vi "ProdaNG.Tree.ProcessStepParams.Add.vi"(5 "Mode":T4, 6 "FileContent":T1, 7 "TestStepsTree":refnum<vi>, 8 "error in (no error)":errorcluster, 9 "units":T5[](array[typedef]), 10 "processStepId":i32, 11 "dbHandleIn":i32) -> (0 "error out":errorcluster, 1 "#changes":i32, 3 "dbHandle":i32)   [LabVIEW 2016]
doc: "This function returns a product structure for a product, which is identified by a part and a serial number.\nImportant information: The field 'individual' was taken over from the field 'allgemein' of the legacy data directly. Because of this most products have the value 0 further on and only a few the value 1. \nParameter:\nhandle is an Integer, which is returned by the function Login() at the creation of a new connection.\nwabcoPartId is the Id of the part.\nserialNumber is the serial number of the product for the part above.\nproduct is a pointer on a product structure, which is filled if the returncode is 0. The structure must be defined in the calling program.\n\nReturncodes:\n0 No error\n< 0 ORACLE Error code\n6 (ERROR_INVALID_HANDLE) in case of an invalid handle\n1403 Record does not exist"
uses:
  Controls/ProdaNG.UnitSimple.ctl
  ProdaNG.Tree.TestViewMode.ctl
  ProdaNG.File.Sequence.ctl
  ProdaNG.Tree.Fglb.Value.ctl
  ProdaNG.File.Step.ctl
  ProdaNG.Tree.Fglb.Data.ctl
  ProdaNG.Tree.Fglb.Element.ctl
  ProdaNG.Tree.Fglb.Action.ctl
  ProdaNG.Configurator.Glb.vi
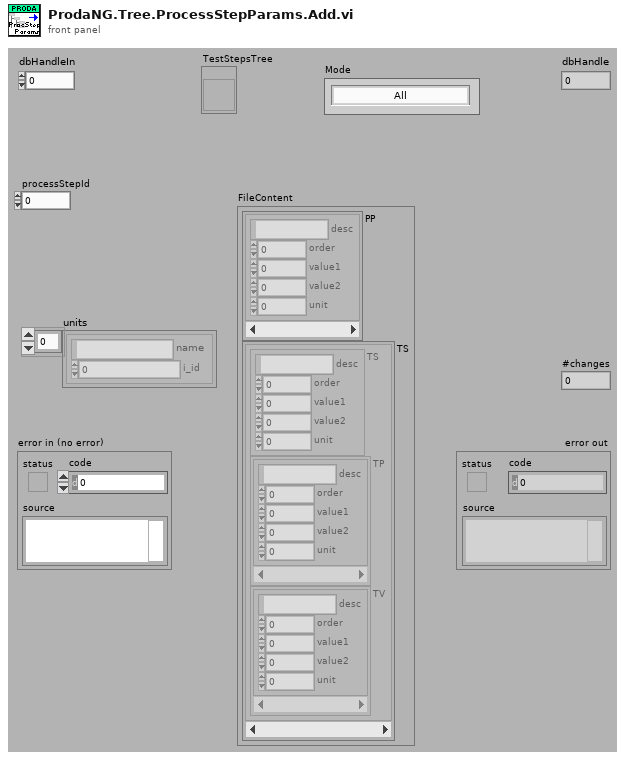
[diagram p1: front panel]
types:
  T1 = typedef "ProdaNG.File.Sequence.ctl" = cluster{"PP":T2[], "TS":T3[]}
  T2 = typedef "ProdaNG.Tree.Fglb.Value.ctl" = cluster{"desc":string, "order":i32, "value1":dbl, "value2":dbl, "unit":i32}
  T3 = typedef "ProdaNG.File.Step.ctl" = cluster{"TS":T2, "TP":T2[], "TV":T2[]}
  T4 = typedef "ProdaNG.Tree.TestViewMode.ctl" = enum16{"All", "Released", "Unreleased"}
  T5 = typedef "ProdaNG.UnitSimple.ctl" = cluster{"name":string, "i_id":i32}
  T6 = typedef "ProdaNG.Tree.Fglb.Action.ctl" = enum16{"init", "add", "get by row", "get by tag", "get by idx"}
  T7 = typedef "ProdaNG.Tree.Fglb.Element.ctl" = enum16{"-", "PP", "TS", "TP", "TV"}
  T8 = typedef "ProdaNG.Tree.Fglb.Data.ctl" = cluster{"tag":string, "row":i32, "element":T7, "idx1":i32, "idx2":i32, "file":bool}
  T9 = typedef "ProdaNG.ProcessStepParam.ctl" = cluster{"i_id":i32, "processStepId":i32, "unitId":i32, "contentId":string, "previewId":string, "value":dbl, "valueText":string, "paramSequence":i32, "history":i32, "mdReason":string, "mdUser":string, "mdTime":string, "description":string}
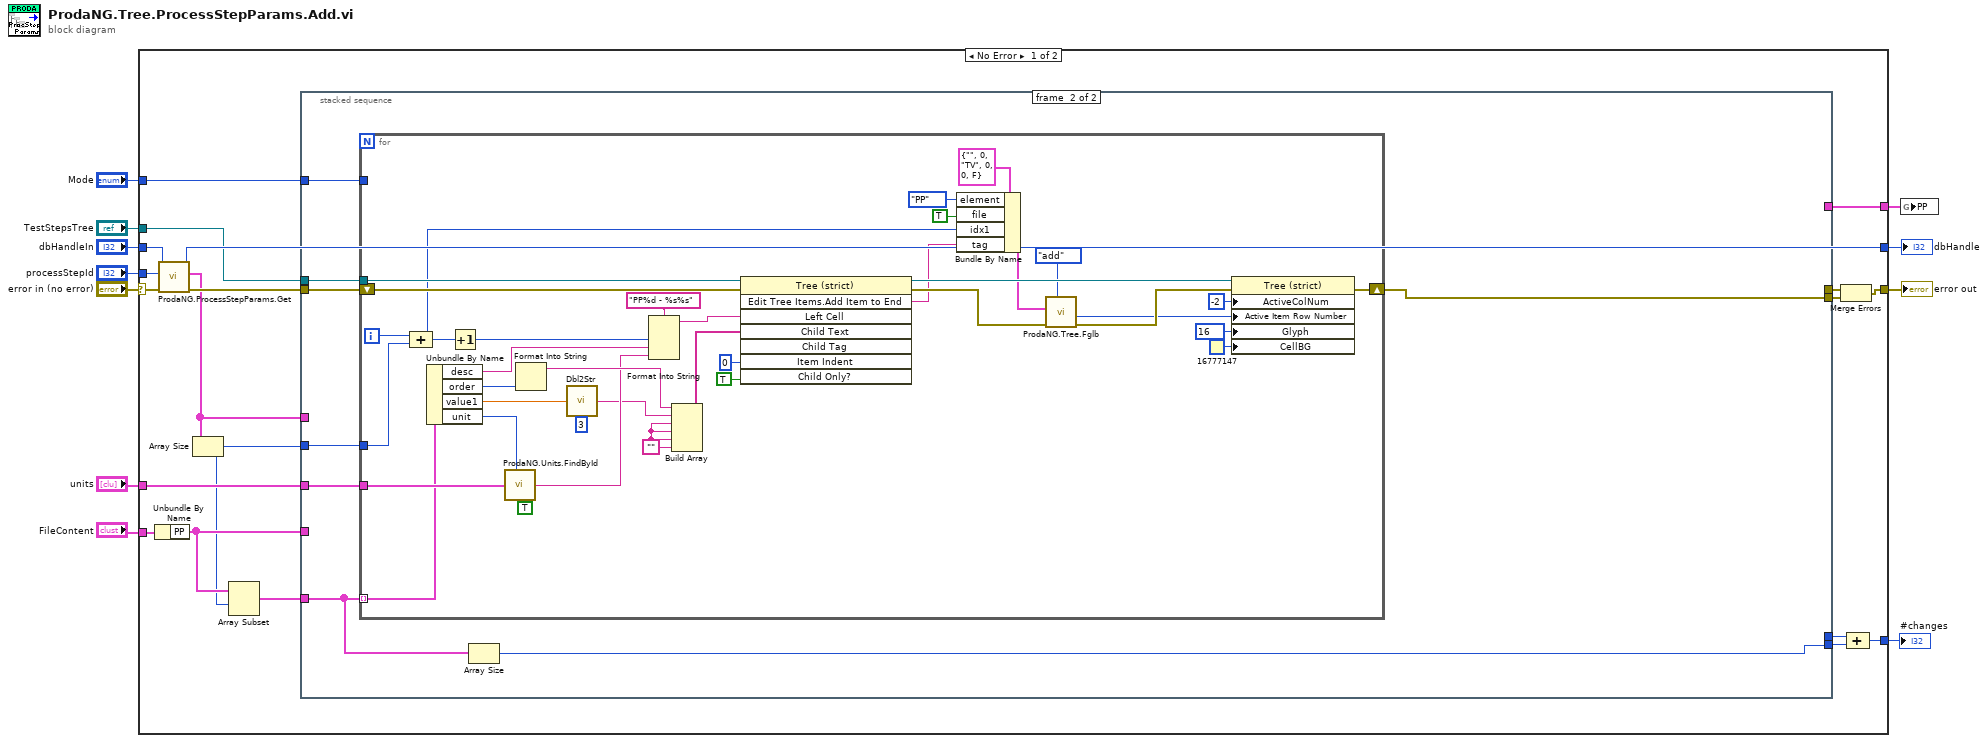
[diagram p0: block diagram]
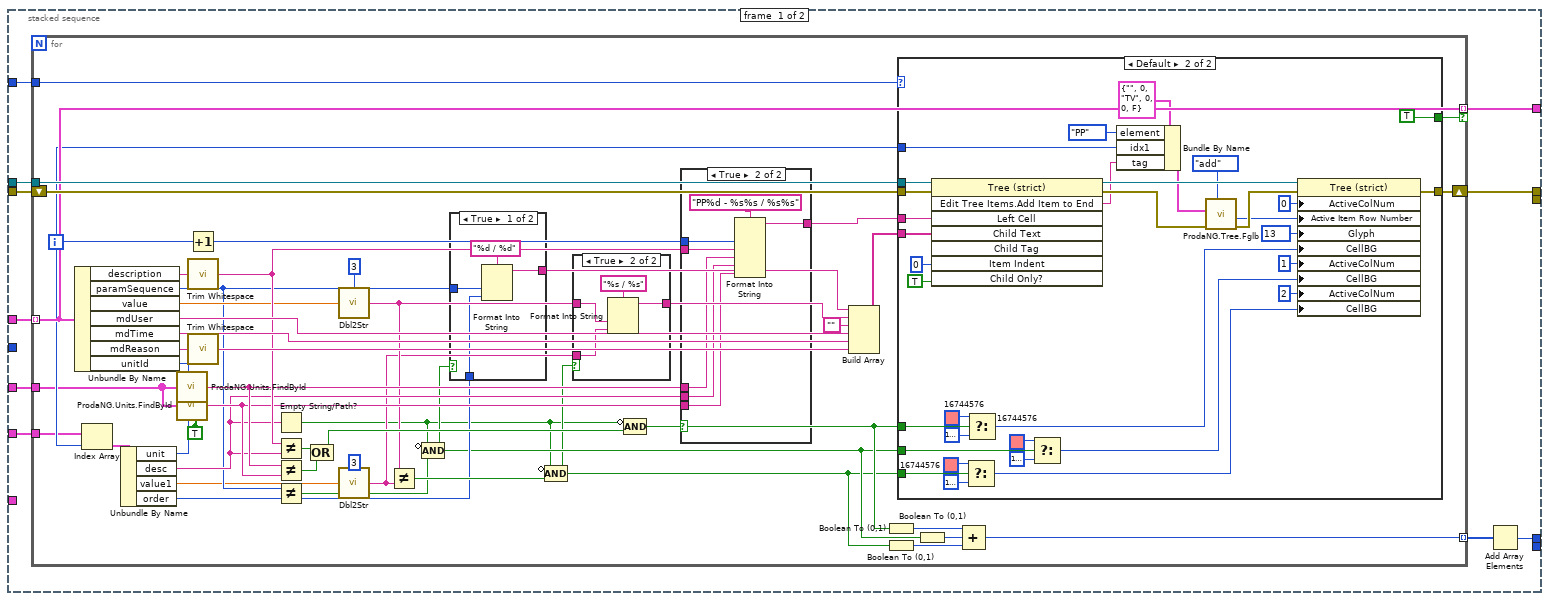
[diagram p2: hidden frame]
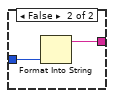
[diagram p3: hidden frame]
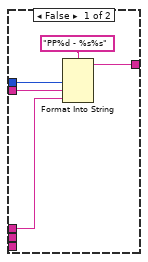
[diagram p5: hidden frame]
diagram:
  n1 = case shown="No Error" "error in (no error)" {
    selector: "error in (no error)" -> [w31 w195]
    tunnel: [w17 w195] -> w10
    tunnel: "dbHandleIn" -> [w29 w194]
    tunnel: [w27 w194] -> w8
    tunnel: "processStepId" -> [w30 _]
    tunnel: "TestStepsTree" -> [w25 _]
    tunnel: "units" -> [w21 _]
    tunnel: "Mode" -> [w24 _]
    tunnel: [w23 _] -> w4
    tunnel: "FileContent" -> [w22 _]
    tunnel: [w14 _] -> w1
    frame No Error {
      n2 = Unbundle By Name(w22) -> ("PP"=w20:T2[])
      n3 = call "ProdaNG.ProcessStepParams.Get.vi"("error in (no error)"=w31, "processStepId"=w30, "dbHandleIn"=w29) -> ("error out"=w26:errorcluster, "ProcStepParams"=w19:T9[], "dbHandle"=w27:i32)  [unwired: 6 in]
      n4 = Array Size(array=w19) -> (size(s)=w12:i32)
      n5 = Array Subset(array=w20, index=w12) -> (w18:T2[])  [unwired: 1 in]
      n6 = stacked-sequence {
        tunnel: [w41 _] -> w28
        tunnel: w26 -> [w40 w156]
        tunnel: w25 -> [w39 w155]
        tunnel: w24 -> [w38 w154]
        tunnel: [w37 _] -> w23
        tunnel: w21 -> [w36 w153]
        tunnel: w20 -> [w35 _]
        tunnel: w19 -> [w34 _]
        tunnel: w18 -> [_ w150]
        tunnel: w12 -> [_ w151]
        tunnel: [_ w152] -> w16
        tunnel: [w33 _] -> w15
        tunnel: [_ w149] -> w13
        frame #0 {
          n7 = for {
            shift-right: [w82] -> w41
            shift-left: w40 -> [w90]
            tunnel: w34 -> [w77] mode=indexing
            tunnel: w39 -> [w86]
            tunnel: w38 -> [w79]
            tunnel: [w77] -> w37 mode=indexing if=w76
            tunnel: w36 -> [w66]
            tunnel: w35 -> [w73]
            tunnel: [w43] -> w32 mode=indexing
            i -> [w74]
            w42 = TRUE
            n8 = Unbundle By Name(w77) -> ("description"=w75:string, "paramSequence"=w59:i32, "value"=w62:dbl, "mdUser"=w88:string, "mdTime"=w89:string, "mdReason"=w85:string, "unitId"=w68:i32)
            n9 = Index Array(array=w73, index=w74) -> (element=w72:T2)
            n10 = Unbundle By Name(w72) -> ("unit"=w67:i32, "desc"=w61:string, "value1"=w53:dbl, "order"=w57:i32)
            n11 = call "ProdaNG.Units.FindById.vi"("units"=w66, "unit id"=w68, "add brackets (F)"=w42) -> ("unit str"=w65:string)
            n12 = call "ProdaNG.Units.FindById.vi"("units"=w66, "unit id"=w67, "add brackets (F)"=w42) -> ("unit str"=w64:string)
            n13 = Increment(x=w74) -> (x+1=w83:i32)
            n14 = call <vilib>:"Trim Whitespace.vi"("string"=w75) -> ("trimmed string"=w71:string)  [unwired: 1 in]
            n15 = call <vilib>:"Trim Whitespace.vi"("string"=w85) -> ("trimmed string"=w81:string)  [unwired: 1 in]
            n16 = Empty String/Path?(string/path=w61) -> (empty?=w44:bool)
            n17 = Not Equal?(x=w71, y=w61) -> (x != y?=w70:bool)
            n18 = Not Equal?(x=w65, y=w64) -> (x != y?=w69:bool)
            n19 = Not Equal?(x=w59, y=w57) -> (x != y?=w58:bool)
            n20 = Compound Arithmetic op=OR(w70, w69) -> (w63:bool)
            n21 = call "Dbl2Str.vi"("Numeric"=w62, "precision (6)"=i16 3) -> ("string"=w55:string)
            n22 = call "Dbl2Str.vi"("Numeric"=w53, "precision (6)"=i16 3) -> ("string"=w52:string)
            n23 = Not Equal?(x=w55, y=w52) -> (x != y?=w60:bool)
            n24 = Compound Arithmetic op=AND(invert w44, w58) -> (w46:bool)
            n25 = case shown="True" w46 {
              tunnel: w59 -> [w94 w96]
              tunnel: [w93 w95] -> w80
              tunnel: w57 -> [w91 _]
              frame True {
                n26 = Format Into String(format string="%d / %d", w94, w91) -> (resulting string=w93:string)  [unwired: 2 in, 1 out]
              }
              frame False {
                n27 = Format Into String(w96) -> (resulting string=w95:string)  [unwired: 3 in, 1 out]
              }
            }
            n28 = Compound Arithmetic op=AND(invert w44, w60) -> (w45:bool)
            n29 = case shown="True" w45 {
              tunnel: [w97 w100] -> w84
              tunnel: w55 -> [w97 w99]
              tunnel: w52 -> [_ w98]
              frame False {
              }
              frame True {
                n30 = Format Into String(format string="%s / %s", w99, w98) -> (resulting string=w100:string)  [unwired: 2 in, 1 out]
              }
            }
            n31 = Compound Arithmetic op=AND(invert w44, w63) -> (w47:bool)
            n32 = case shown="True" w47 {
              tunnel: w65 -> [w102 w109]
              tunnel: w83 -> [w105 w112]
              tunnel: w71 -> [w104 w111]
              tunnel: [w103 w110] -> w78
              tunnel: w61 -> [_ w108]
              tunnel: w64 -> [_ w107]
              frame False {
                n33 = Format Into String(format string="PP%d - %s%s", w105, w104, w102) -> (resulting string=w103:string)  [unwired: 2 in, 1 out]
              }
              frame True {
                n34 = Format Into String(format string="PP%d - %s%s / %s%s", w112, w111, w109, w108, w107) -> (resulting string=w110:string)  [unwired: 2 in, 1 out]
              }
            }
            n35 = Build Array(w80, w84, "", w88, w89, w81) -> (w87:string[])
            n36 = Boolean To (0,1)(Boolean=w47) -> (0, 1=w50:i16)
            n37 = Boolean To (0,1)(Boolean=w45) -> (0, 1=w48:i16)
            n38 = case shown="Default" w79 {
              tunnel: w90 -> [w114 w146]
              tunnel: w78 -> [_ w145]
              tunnel: w87 -> [_ w144]
              tunnel: w86 -> [_ w143]
              tunnel: [w114 w137] -> w82
              tunnel: w74 -> [_ w134]
              tunnel: [_ TRUE] -> w76
              tunnel: w47 -> [_ w128]
              tunnel: w46 -> [_ w122]
              tunnel: w45 -> [_ w117]
              frame "Unreleased" {
              }
              frame Default {
                n39 = invoke on="Invoke Node" class="Tree (strict)" method="Edit Tree Items.Add Item to End"(reference=w143, error in=w146, "Left Cell"=w145, "Child Text"=w144, "Item Indent"=0 ("New Item Indentation"), "Child Only?"=TRUE) -> (reference out=w139:refnum<vi>, error out=w132:errorcluster, "Edit Tree Items:Add Item to End"=w129:string)  [unwired: 2 in, 5 out]
                n40 = Select(t=u32 16744576, s=w117, f=u32 16777225) -> (s? t:f=w116:u32)
                n41 = Select(t=u32 16744576, s=w128, f=u32 16777225) -> (s? t:f=w115:u32)
                n42 = Select(t=u32 16744576, s=w122, f=u32 16777225) -> (s? t:f=w121:u32)
                n43 = Bundle By Name(cluster=T8 {"tag"="", "row"=0, "element"=enum."TV", "idx1"=0, "idx2"=0, "file"=FALSE} ("entry in"), "element"=ProdaNG.Tree.Fglb.Element."PP", "idx1"=w134, "tag"=w129) -> (w133:T8)
                n44 = call "ProdaNG.Tree.Fglb.vi"("Action (add)"=ProdaNG.Tree.Fglb.Action."add", "error in"=w132, "entry in"=w133) -> ("error out"=w140:errorcluster, "active row"=w138:i32)  [unwired: 6 in, 1 out]
                n45 = property class="Tree (strict)"(reference=w139, error in=w140, "ActiveColNum"=0 ("Active Cell:Active Column Number"), "Active Item Row Number"=w138, "Glyph"=13, "CellBG"=w115, "ActiveColNum"=1 ("Active Cell:Active Column Number"), "CellBG"=w121, "ActiveColNum"=2 ("Active Cell:Active Column Number"), "CellBG"=w116) -> (error out=w137:errorcluster)  [unwired: 1 out]
              }
            }
            n46 = Boolean To (0,1)(Boolean=w46) -> (0, 1=w49:i16)
            n47 = Compound Arithmetic op=ADD(w50, w49, w48) -> (w43:i16)
          }
          n48 = Add Array Elements(numeric array=w32) -> (sum=w33:i16)
        }
        frame #1 {
          n49 = for {
            shift-right: [w189] -> w152
            shift-left: w156 -> [w193]
            tunnel: w155 -> [w191]
            tunnel: w154 -> [_]
            tunnel: w153 -> [w183]
            tunnel: w150 -> [w175] mode=indexing
            tunnel: w151 -> [w172]
            i -> [w185]
            w161 = ""
            n50 = Compound Arithmetic op=ADD(w185, w172) -> (w164:i32)
            n51 = Unbundle By Name(w175) -> ("desc"=w186:string, "order"=w181:i32, "value1"=w160:dbl, "unit"=w184:i32)
            n52 = Increment(x=w164) -> (x+1=w190:i32)
            n53 = call "ProdaNG.Units.FindById.vi"("units"=w183, "unit id"=w184, "add brackets (F)"=TRUE ("add quotas (F)")) -> ("unit str"=w182:string)
            n54 = Format Into String(w181) -> (resulting string=w188:string)  [unwired: 3 in, 1 out]
            n55 = call "Dbl2Str.vi"("Numeric"=w160, "precision (6)"=i16 3) -> ("string"=w159:string)
            n56 = Format Into String(format string="PP%d - %s%s", w190, w186, w182) -> (resulting string=w187:string)  [unwired: 2 in, 1 out]
            n57 = Build Array(w188, w159, w161, w161, w161, w161) -> (w192:string[])
            n58 = invoke on="Invoke Node" class="Tree (strict)" method="Edit Tree Items.Add Item to End"(reference=w191, error in=w193, "Left Cell"=w187, "Child Text"=w192, "Item Indent"=0 ("New Item Indentation"), "Child Only?"=TRUE) -> (reference out=w176:refnum<vi>, error out=w168:errorcluster, "Edit Tree Items:Add Item to End"=w165:string)  [unwired: 2 in, 5 out]
            n59 = Bundle By Name(cluster=T8 {"tag"="", "row"=0, "element"=enum."TV", "idx1"=0, "idx2"=0, "file"=FALSE} ("entry in"), "element"=ProdaNG.Tree.Fglb.Element."PP", "file"=TRUE, "idx1"=w164, "tag"=w165) -> (w166:T8)
            n60 = call "ProdaNG.Tree.Fglb.vi"("Action (add)"=ProdaNG.Tree.Fglb.Action."add", "error in"=w168, "entry in"=w166) -> ("error out"=w167:errorcluster, "active row"=w162:i32)  [unwired: 6 in, 1 out]
            n61 = property class="Tree (strict)"(reference=w176, error in=w167, "ActiveColNum"=-2 ("Active Cell:Active Column Number"), "Active Item Row Number"=w162, "Glyph"=16, "CellBG"=u32 16777147) -> (error out=w189:errorcluster)  [unwired: 1 out]
          }
          n62 = Array Size(array=w150) -> (size(s)=w149:i32)
        }
      }
      n63 = Merge Errors(w28, w16) -> (w17:errorcluster)
      n64 = Compound Arithmetic op=ADD(w15, w13) -> (w14:i32)
    }
    frame Error {
    }
  }
  "error out" <- w10
  "dbHandle" <- w8
  "#changes" <- w1
  n65 = global write "ProdaNG.Configurator.Glb.vi" "PP"(w4) -> ()
